vi "IV 023.vi"() -> ()   [LabVIEW 2021]
panel:
  in  "L3":dbl(slide) scale=0.0..1.0
  in  "P3":dbl(knob) scale=0.0..360.0
  in  "P2":dbl(knob) scale=0.0..360.0
  out "XY Graph":cluster{dbl[], dbl[]}(graph)
  in  "L2":dbl(slide) scale=0.0..1.0
  in  "L1":dbl(slide) scale=0.0..1.0
  in  "P1":dbl(knob) scale=0.0..360.0
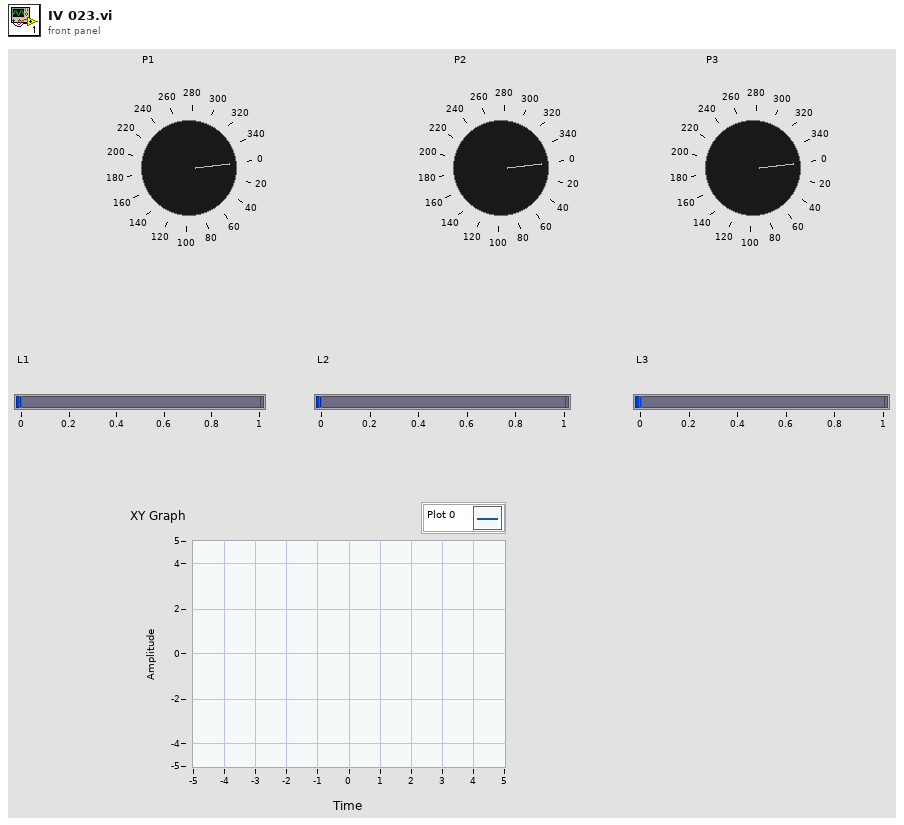
[diagram p1: front panel]
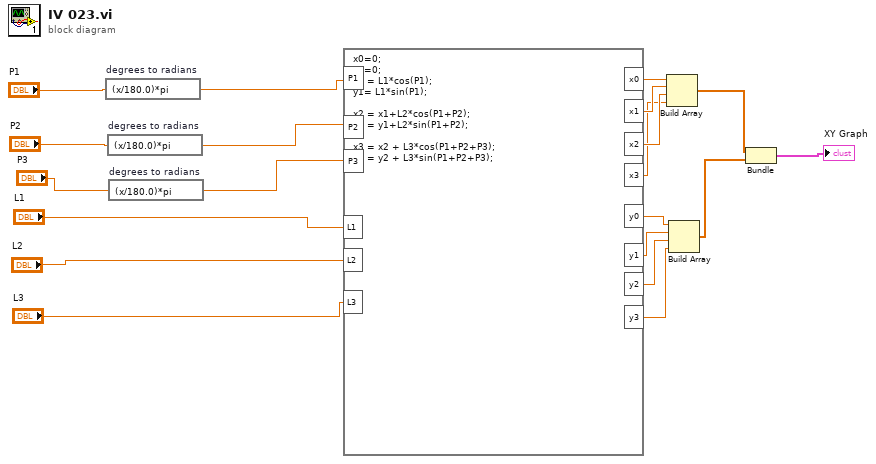
[diagram p0: block diagram]
diagram:
  n1 = expression code="(x/180.0)*pi" "degrees to radians"("P1") -> (w19:dbl)
  n2 = expression code="(x/180.0)*pi" "degrees to radians"("P2") -> (w6:dbl)
  n3 = expression code="(x/180.0)*pi" "degrees to radians"("P3") -> (w2:dbl)
  n4 = formula code="x0=0;\ny0=0;\nx1 = L1*cos(P1);\ny1= L1*sin(P1);\n\nx2 = x1+L2*cos(P1+P2);\ny2 = y1+L2*sin(P1+P2);\n\nx3 = x2 + L3*cos(P1+P2+P3);\nx3 = y2 + L3*sin(P1+P2+P3);"("P1"=w19, "L1"="L1", "L2"="L2", "P2"=w6, "L3"="L3", "P3"=w2) -> ("x0"=w17:dbl, "y0"=w15:dbl, "x1"=w16:dbl, "y1"=w14:dbl, "x2"=w8:dbl, "y2"=w7:dbl, "x3"=w4:dbl, "y3"=w5:dbl)
  n5 = Build Array(w17, w16, w8, w4) -> (w13:dbl[])
  n6 = Build Array(w15, w14, w7, w5) -> (w12:dbl[])
  n7 = Bundle(w13, w12) -> (→"XY Graph":cluster{dbl[], dbl[]})  [unwired: 1 in]
